vi "Motor Begin.vi"(8 "error in (no error)":errorcluster) -> (0 "error out":errorcluster)   [LabVIEW 2013]
uses:
  <vilib>/Rock Robotics/SystemInterfaces/DIO/FPGA_DIOPWMChannel.ctl
  <vilib>/Rock Robotics/WPI/MotorControl/WPI_MotorControlOpen Talon.vi
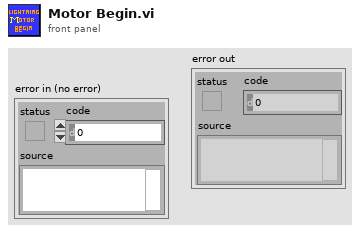
[diagram p1: front panel]
types:
  T1 = typedef "FPGA_DIOPWMChannel.ctl" = enum8{"PWM 1", "PWM 2", "PWM 3", "PWM 4", "PWM 5", "PWM 6", "PWM 7", "PWM 8", "PWM 9", "PWM 10", "Invalid"}
  T2 = typedef "WPI_MotorControlDeviceRef.ctl" = cluster{"DeviceStatus":errorcluster, "Type":enum16{"PWM", "CAN"}, "PWM":cluster{"Digital Module":T3, "PWM Channel":T1, "DeadBand":T4}, "CAN":cluster{"Device Number":u8, "Control Mode":T5, "Semaphore":T6, "Max Vout":dbl}, "Invert":bool, "TransformRef":T7, "InvTransformRef":T7}
  T3 = typedef "FPGA_TypedefDigitalModule.ctl" = enum16{"Digital Module 1", "Digital Module 2"}
  T4 = typedef "WPI_PWMDeadband.ctl" = cluster{"Name":string, "maxPositivePwm":i32, "minPositivePwm":i32, "centerPwm":i32, "maxNegativePwm":i32, "minNegativePwm":i32, "angularRange":u16}
  T5 = typedef "WPI_CANJaguar_ControlMode.ctl" = enum8{"Percent VBus", "Current", "Speed", "Position", "Voltage"}
  T6 = typedef "Semaphore RefNum" = refnum<k1>
  T7 = typedef "WPI_PWMTransform_ConPane.ctl" = refnum<vi>
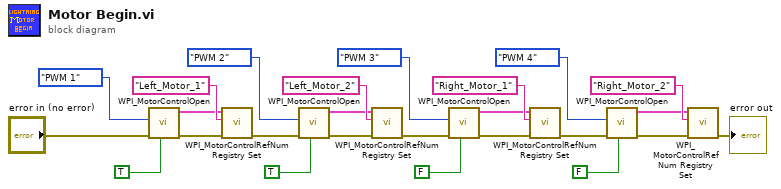
[diagram p0: block diagram]
diagram:
  n1 = call-poly <vilib>:"WPI_MotorControlOpen.vi"("Invert"=TRUE, "error in (no error)"="error in (no error)", "PWM Channel"=FPGA_DIOPWMChannel."PWM 1") -> ("error out"=w19:errorcluster, "MotorControlDeviceRef"=w15:T2)  [unwired: 7 in]
  n2 = call <vilib>:"WPI_MotorControlRefNum Registry Set.vi"("error in (no error)"=w19, "refnum name"="Left_Motor_1", "MotorControlDevRef"=w15) -> ("error out"=w25:errorcluster)  [unwired: 7 in, 1 out]
  n3 = call-poly <vilib>:"WPI_MotorControlOpen.vi"("Invert"=TRUE, "error in (no error)"=w25, "PWM Channel"=FPGA_DIOPWMChannel."PWM 2") -> ("error out"=w24:errorcluster, "MotorControlDeviceRef"=w21:T2)  [unwired: 7 in]
  n4 = call <vilib>:"WPI_MotorControlRefNum Registry Set.vi"("error in (no error)"=w24, "refnum name"="Left_Motor_2", "MotorControlDevRef"=w21) -> ("error out"=w9:errorcluster)  [unwired: 7 in, 1 out]
  n5 = call-poly <vilib>:"WPI_MotorControlOpen.vi"("Invert"=FALSE, "error in (no error)"=w9, "PWM Channel"=FPGA_DIOPWMChannel."PWM 3") -> ("error out"=w10:errorcluster, "MotorControlDeviceRef"=w1:T2)  [unwired: 7 in]
  n6 = call <vilib>:"WPI_MotorControlRefNum Registry Set.vi"("error in (no error)"=w10, "refnum name"="Right_Motor_1", "MotorControlDevRef"=w1) -> ("error out"=w4:errorcluster)  [unwired: 7 in, 1 out]
  n7 = call-poly <vilib>:"WPI_MotorControlOpen.vi"("Invert"=FALSE, "error in (no error)"=w4, "PWM Channel"=FPGA_DIOPWMChannel."PWM 4") -> ("error out"=w5:errorcluster, "MotorControlDeviceRef"=w2:T2)  [unwired: 7 in]
  n8 = call <vilib>:"WPI_MotorControlRefNum Registry Set.vi"("error in (no error)"=w5, "refnum name"="Right_Motor_2", "MotorControlDevRef"=w2) -> ("error out"=→"error out":errorcluster)  [unwired: 7 in, 1 out]
